vi "DrivePropertiesConvert.vi"(4 "Position Offset In":dbl, 5 "Channel Properties In":T1={"Channel Name"="", "Vel. Default"=5.0, "Acc. Default"=5.0, "Vel. Max"=5.0, "Vel. Min"=5.0, "Acc. Max"=5.0, "Acc. Min"=5.0, "Pulses/unit"=0.0, "Address"=0, "Pulse Offset"=0, "Pos Tolerance"=0.0, "Pulses/rev"=0.0, "Backlash/Eng units"=0.0, "Current Pos"=0.0, "Ch Status"=enum."Active", "Port Name"="", "Axis Transform mode"="", "Metadata Ch Name"="", "Type"=""} {"Current Pos" format="%.2f"; "Backlash/Eng units" format="%.2f"; "Pulses/rev" format="%.2f"; "Pos Tolerance" format="%.2f"; "Pulses/unit" format="%.2f"; "Acc. Min" format="%.2f"; "Acc. Max" format="%.2f"; "Vel. Min" format="%.2f"; "Vel. Max" format="%.2f"; "Acc. Default" format="%.2f"; "Vel. Default" format="%.2f"}, 6 "String in":string[](array[string]), 7 "Ch names In":string[](array[string]), 8 "Mode":enum16{"Cluster to String", "String to Cluster"}(ring)) -> (0 "Channel Properties Out":T1={"Channel Name"="", "Vel. Default"=5.0, "Acc. Default"=5.0, "Vel. Max"=5.0, "Vel. Min"=5.0, "Acc. Max"=5.0, "Acc. Min"=5.0, "Pulses/unit"=0.0, "Address"=0, "Pulse Offset"=0, "Pos Tolerance"=0.0, "Pulses/rev"=0.0, "Backlash/Eng units"=0.0, "Current Pos"=0.0, "Ch Status"=enum."Active", "Port Name"="", "Axis Transform mode"="", "Metadata Ch Name"="", "Type"=""} {"Current Pos" format="%.2f"; "Backlash/Eng units" format="%.2f"; "Pulses/rev" format="%.2f"; "Pos Tolerance" format="%.2f"; "Pulses/unit" format="%.2f"; "Acc. Min" format="%.2f"; "Acc. Max" format="%.2f"; "Vel. Min" format="%.2f"; "Vel. Max" format="%.2f"; "Acc. Default" format="%.2f"; "Vel. Default" format="%.2f"}, 1 "String Values":string[](array[string]), 2 "Ch names":string[](array[string]), 3 "Position Offset Out":dbl)   [LabVIEW 2010]
uses:
  DriveProperties.ctl
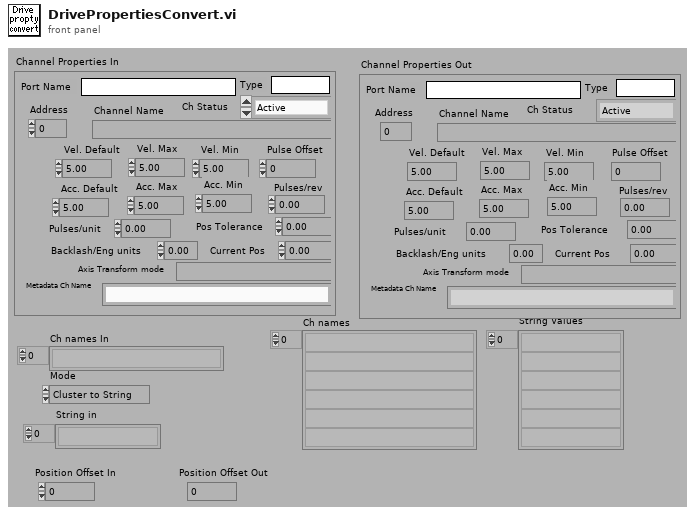
[diagram p1: front panel]
types:
  T1 = typedef "DriveProperties.ctl" = cluster{"Channel Name":string, "Vel. Default":dbl, "Acc. Default":dbl, "Vel. Max":dbl, "Vel. Min":dbl, "Acc. Max":dbl, "Acc. Min":dbl, "Pulses/unit":dbl, "Address":u8, "Pulse Offset":i32, "Pos Tolerance":dbl, "Pulses/rev":dbl, "Backlash/Eng units":dbl, "Current Pos":dbl, "Ch Status":enum16{"Active", "Offline", "Simulate"}, "Port Name":string, "Axis Transform mode":string, "Metadata Ch Name":string, "Type":string}
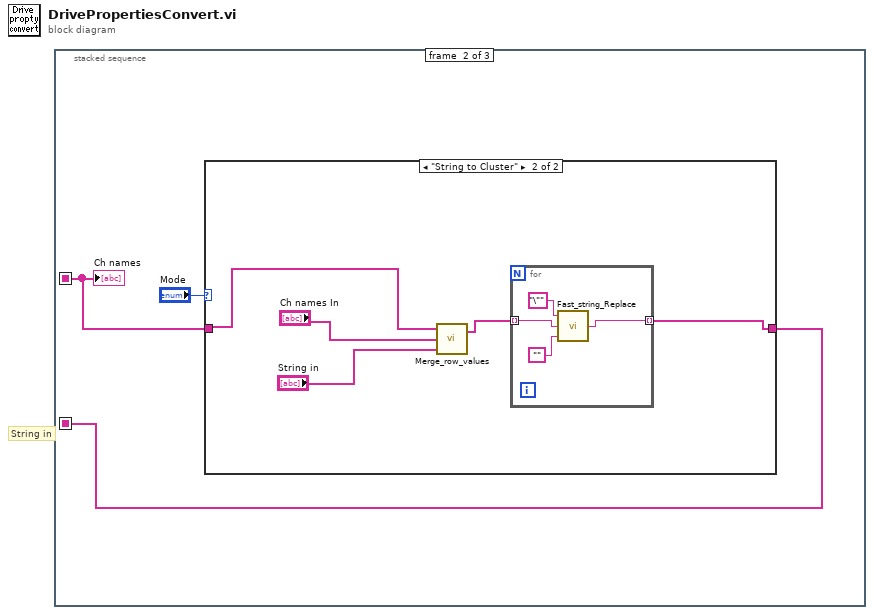
[diagram p0: block diagram]
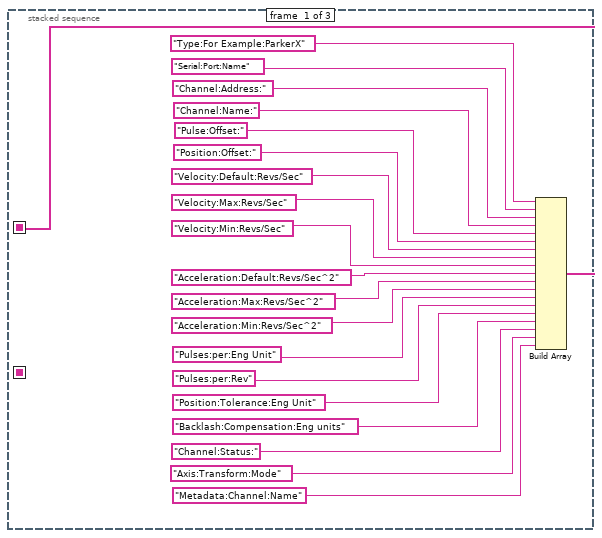
[diagram p2: hidden frame]
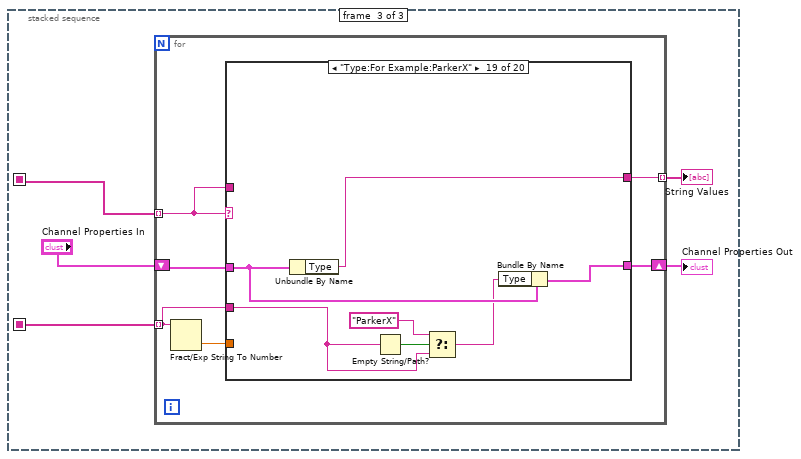
[diagram p4: hidden frame]
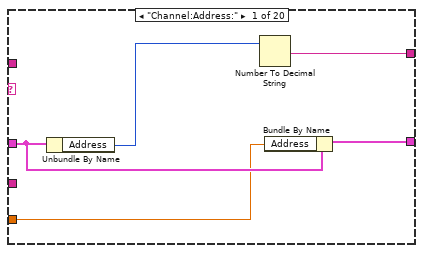
[diagram p5: hidden frame]
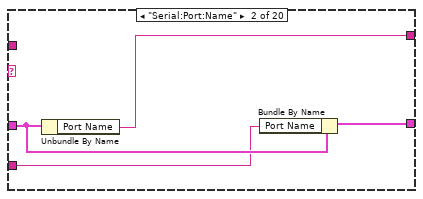
[diagram p6: hidden frame]
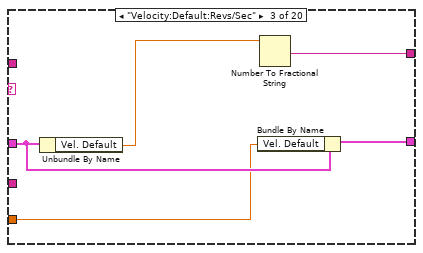
[diagram p7: hidden frame]
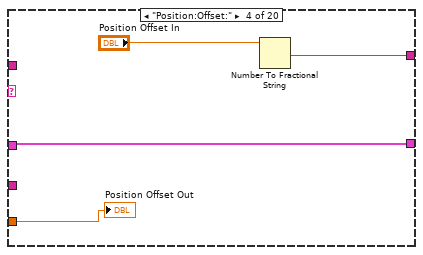
[diagram p8: hidden frame]
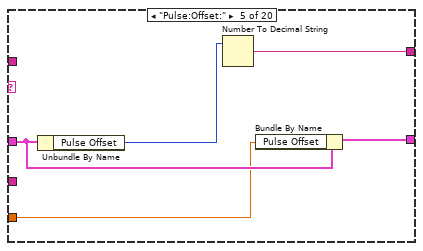
[diagram p9: hidden frame]
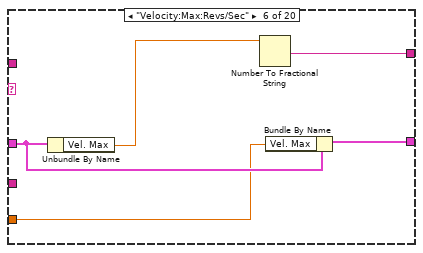
[diagram p10: hidden frame]
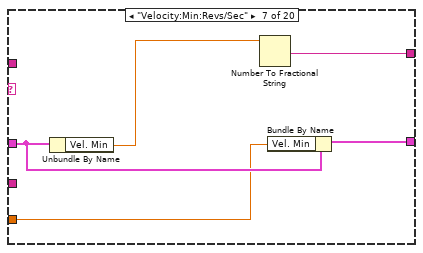
[diagram p11: hidden frame]
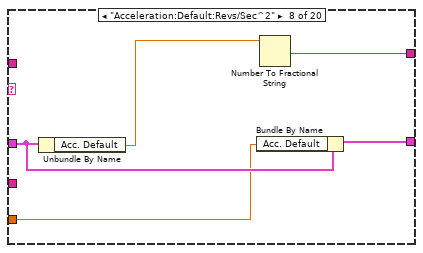
[diagram p12: hidden frame]
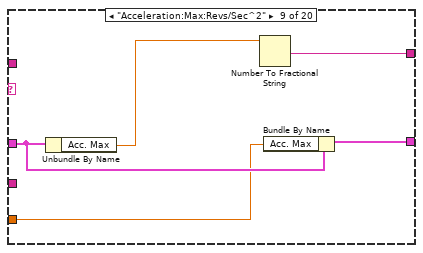
[diagram p13: hidden frame]
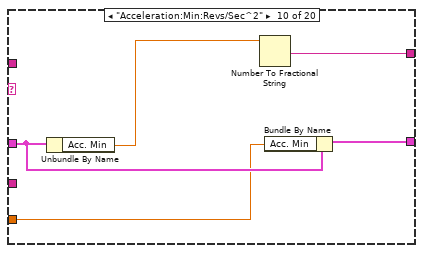
[diagram p14: hidden frame]
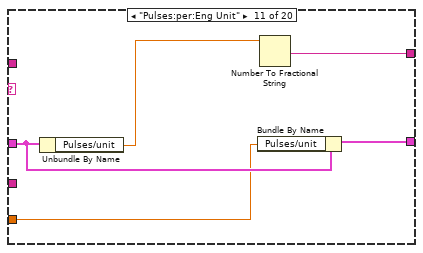
[diagram p15: hidden frame]
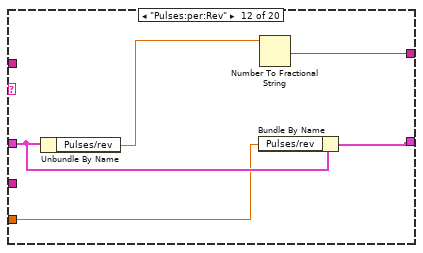
[diagram p16: hidden frame]
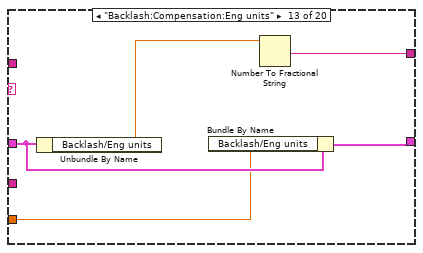
[diagram p17: hidden frame]
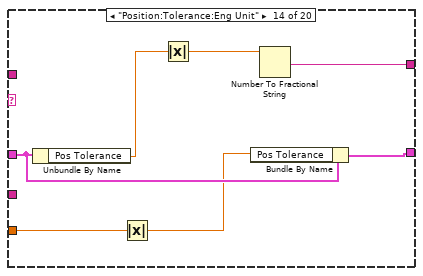
[diagram p18: hidden frame]
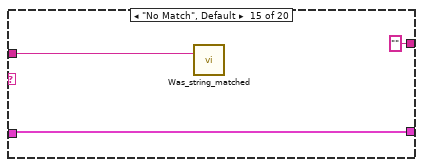
[diagram p19: hidden frame]
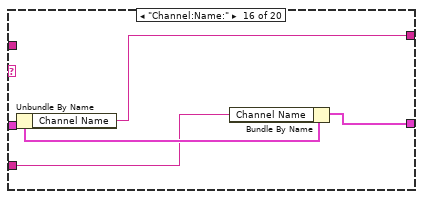
[diagram p20: hidden frame]
diagram:
  # "String in"
  n1 = stacked-sequence {
    seq-local: [w11 _ _] -> [_ w22 w38]
    seq-local: [_ w21 _] -> [_ _ w37]
    frame #0 {
      n2 = Build Array("Type:For Example:ParkerX", "Serial:Port:Name", "Channel:Address:", "Channel:Name:", "Pulse:Offset:", "Position:Offset:", "Velocity:Default:Revs/Sec", "Velocity:Max:Revs/Sec", "Velocity:Min:Revs/Sec", "Acceleration:Default:Revs/Sec^2", "Acceleration:Max:Revs/Sec^2", "Acceleration:Min:Revs/Sec^2", "Pulses:per:Eng Unit", "Pulses:per:Rev", "Position:Tolerance:Eng Unit", "Backlash:Compensation:Eng units", "Channel:Status:", "Axis:Transform:Mode", "Metadata:Channel:Name") -> (w11:string[])
    }
    frame #1 {
      n3 = case shown="\"String to Cluster\"" "Mode" {
        tunnel: [w24 w25] -> w21
        tunnel: w22 -> [w24 w27]
        frame "Cluster to String" {
        }
        frame "String to Cluster" {
          n4 = call "Merge_row_values.vi"("Present Row values"="String in", "Present Channels"="Ch names In", "Desired Channels"=w27) -> ("Desired Row values"=w26:string[])  [unwired: 1 out]
          n5 = for {
            tunnel: w26 -> [w33] mode=indexing
            tunnel: [w32] -> w25 mode=indexing
            n6 = call "Fast_string_Replace.vi"("Replace match with:"="", "Input String"=w33, "regular expression"="\"") -> ("Output String"=w32:string)  [unwired: 2 out]
          }
        }
      }
      "Ch names" <- w22
    }
    frame #2 {
      n7 = for {
        tunnel: w38 -> [w41] mode=indexing
        tunnel: w37 -> [w44] mode=indexing
        tunnel: [w42] -> w36 mode=indexing
        shift-right: [w39] -> w34
        shift-left: "Channel Properties In" -> [w40]
        n8 = Fract/Exp String To Number(string=w44) -> (number=w43:dbl)  [unwired: 4 out]
        n9 = case shown="\"Type:For Example:ParkerX\"" w41 {
          tunnel: w40 -> [w49 w53 w58 w60 w67 w72 w77 w82 w87 w92 w97 w102 w107 w114 w115 w120 w124 w128 w135 w142]
          tunnel: w44 -> [_ w51 _ _ _ _ _ _ _ _ _ _ _ _ _ w119 w123 w127 w131 w138]
          tunnel: [w46 w52 w55 w62 w63 w69 w74 w79 w84 w89 w94 w99 w104 w111 "" ("Channel Name") w121 w125 w129 w136 w139] -> w42
          tunnel: w43 -> [w48 _ w57 w59 w66 w71 w76 w81 w86 w91 w96 w101 w106 w113 _ _ _ _ _ _]
          tunnel: w41 -> [_ _ _ _ _ _ _ _ _ _ _ _ _ _ w116 _ _ _ _ _]
          tunnel: [w45 w50 w54 w60 w65 w68 w73 w78 w83 w88 w93 w98 w103 w108 w115 w118 w122 w126 w134 w141] -> w39
          frame "Channel:Address:" {
            n10 = Unbundle By Name(w49) -> ("Address"=w47:u8)
            n11 = Number To Decimal String(number=w47) -> (decimal integer string=w46:string)  [unwired: 1 out]
            n12 = Bundle By Name(cluster=w49, "Address"=w48) -> (w45:T1)
          }
          frame "Serial:Port:Name" {
            n13 = Unbundle By Name(w53) -> ("Port Name"=w52:string)
            n14 = Bundle By Name(cluster=w53, "Port Name"=w51) -> (w50:T1)
          }
          frame "Velocity:Default:Revs/Sec" {
            n15 = Unbundle By Name(w58) -> ("Vel. Default"=w56:dbl)
            n16 = Bundle By Name(cluster=w58, "Vel. Default"=w57) -> (w54:T1)
            n17 = Number To Fractional String(number=w56) -> (F-format string=w55:string)  [unwired: 3 out]
          }
          frame "Position:Offset:" {
            n18 = Number To Fractional String(number="Position Offset In") -> (F-format string=w62:string)  [unwired: 3 out]
            "Position Offset Out" <- w59
          }
          frame "Pulse:Offset:" {
            n19 = Unbundle By Name(w67) -> ("Pulse Offset"=w64:i32)
            n20 = Number To Decimal String(number=w64) -> (decimal integer string=w63:string)  [unwired: 1 out]
            n21 = Bundle By Name(cluster=w67, "Pulse Offset"=w66) -> (w65:T1)
          }
          frame "Velocity:Max:Revs/Sec" {
            n22 = Unbundle By Name(w72) -> ("Vel. Max"=w70:dbl)
            n23 = Number To Fractional String(number=w70) -> (F-format string=w69:string)  [unwired: 3 out]
            n24 = Bundle By Name(cluster=w72, "Vel. Max"=w71) -> (w68:T1)
          }
          frame "Velocity:Min:Revs/Sec" {
            n25 = Unbundle By Name(w77) -> ("Vel. Min"=w75:dbl)
            n26 = Number To Fractional String(number=w75) -> (F-format string=w74:string)  [unwired: 3 out]
            n27 = Bundle By Name(cluster=w77, "Vel. Min"=w76) -> (w73:T1)
          }
          frame "Acceleration:Default:Revs/Sec^2" {
            n28 = Unbundle By Name(w82) -> ("Acc. Default"=w80:dbl)
            n29 = Bundle By Name(cluster=w82, "Acc. Default"=w81) -> (w78:T1)
            n30 = Number To Fractional String(number=w80) -> (F-format string=w79:string)  [unwired: 3 out]
          }
          frame "Acceleration:Max:Revs/Sec^2" {
            n31 = Unbundle By Name(w87) -> ("Acc. Max"=w85:dbl)
            n32 = Number To Fractional String(number=w85) -> (F-format string=w84:string)  [unwired: 3 out]
            n33 = Bundle By Name(cluster=w87, "Acc. Max"=w86) -> (w83:T1)
          }
          frame "Acceleration:Min:Revs/Sec^2" {
            n34 = Unbundle By Name(w92) -> ("Acc. Min"=w90:dbl)
            n35 = Number To Fractional String(number=w90) -> (F-format string=w89:string)  [unwired: 3 out]
            n36 = Bundle By Name(cluster=w92, "Acc. Min"=w91) -> (w88:T1)
          }
          frame "Pulses:per:Eng Unit" {
            n37 = Unbundle By Name(w97) -> ("Pulses/unit"=w95:dbl)
            n38 = Bundle By Name(cluster=w97, "Pulses/unit"=w96) -> (w93:T1)
            n39 = Number To Fractional String(number=w95) -> (F-format string=w94:string)  [unwired: 3 out]
          }
          frame "Pulses:per:Rev" {
            n40 = Unbundle By Name(w102) -> ("Pulses/rev"=w100:dbl)
            n41 = Bundle By Name(cluster=w102, "Pulses/rev"=w101) -> (w98:T1)
            n42 = Number To Fractional String(number=w100) -> (F-format string=w99:string)  [unwired: 3 out]
          }
          frame "Backlash:Compensation:Eng units" {
            n43 = Unbundle By Name(w107) -> ("Backlash/Eng units"=w105:dbl)
            n44 = Bundle By Name(cluster=w107, "Backlash/Eng units"=w106) -> (w103:T1)
            n45 = Number To Fractional String(number=w105) -> (F-format string=w104:string)  [unwired: 3 out]
          }
          frame "Position:Tolerance:Eng Unit" {
            n46 = Unbundle By Name(w114) -> ("Pos Tolerance"=w112:dbl)
            n47 = Absolute Value(x=w113) -> (abs(x)=w109:dbl)
            n48 = Absolute Value(x=w112) -> (abs(x)=w110:dbl)
            n49 = Bundle By Name(cluster=w114, "Pos Tolerance"=w109) -> (w108:T1)
            n50 = Number To Fractional String(number=w110) -> (F-format string=w111:string)  [unwired: 3 out]
          }
          frame "No Match", Default {
            n51 = call "Was_string_matched.vi"("Variable name"=w116) -> ()  [unwired: 2 in]
          }
          frame "Channel:Name:" {
            n52 = Unbundle By Name(w120) -> ("Channel Name"=w121:string)
            n53 = Bundle By Name(cluster=w120, "Channel Name"=w119) -> (w118:T1)
          }
          frame "Axis:Transform:Mode" {
            n54 = Unbundle By Name(w124) -> ("Axis Transform mode"=w125:string)
            n55 = Bundle By Name(cluster=w124, "Axis Transform mode"=w123) -> (w122:T1)
          }
          frame "Metadata:Channel:Name" {
            n56 = Unbundle By Name(w128) -> ("Metadata Ch Name"=w129:string)
            n57 = Bundle By Name(cluster=w128, "Metadata Ch Name"=w127) -> (w126:T1)
          }
          frame "Type:For Example:ParkerX" {
            n58 = Unbundle By Name(w135) -> ("Type"=w136:string)
            n59 = Empty String/Path?(string/path=w131) -> (empty?=w133:bool)
            n60 = Select(t="ParkerX", s=w133, f=w131) -> (s? t:f=w130:string)
            n61 = Bundle By Name(cluster=w135, "Type"=w130) -> (w134:T1)
          }
          frame "Channel:Status:" {
            n62 = Unbundle By Name(w142) -> ("Ch Status"=w140:enum16{"Active", "Offline", "Simulate"})
            n63 = case shown="\"Active\"" w140 {
              tunnel: ["Active" "Simulate" "Offline"] -> w139
              frame "Active" {
              }
              frame "Simulate" {
              }
              frame "Offline" {
              }
            }
            n64 = case shown="\"Active\", Default" w138 {
              tunnel: [enum16{"Active", "Offline", "Simulate"}."Active" ("Ch Status") enum16{"Active", "Offline", "Simulate"}."Simulate" ("Ch Status") enum16{"Active", "Offline", "Simulate"}."Offline" ("Ch Status") enum16{"Active", "Offline", "Simulate"}."Active" ("Ch Status") enum16{"Active", "Offline", "Simulate"}."Offline" ("Ch Status")] -> w137
              frame "Active", Default {
              }
              frame "Simulate" {
              }
              frame "Offline" {
              }
              frame "TRUE" {
              }
              frame "FALSE" {
              }
            }
            n65 = Bundle By Name(cluster=w142, "Ch Status"=w137) -> (w141:T1)
          }
        }
      }
      "Channel Properties Out" <- w34
      "String Values" <- w36
    }
  }
